vi "CT_SaveMultiWaveformWithNames.vi"(1 "error in (no error)":errorcluster, 2 "delimiter (Tab)":string="\t", 3 "waveforms":waveform(dbl)[][](array[waveform]), 4 "file path (dialog if empty)":path) -> (0 "error out":errorcluster)   [LabVIEW 2009]
panel:
  out "spreadsheet string":string
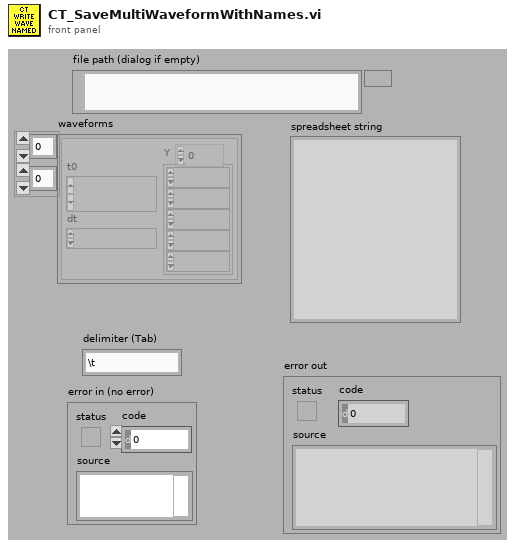
[diagram p1: front panel]
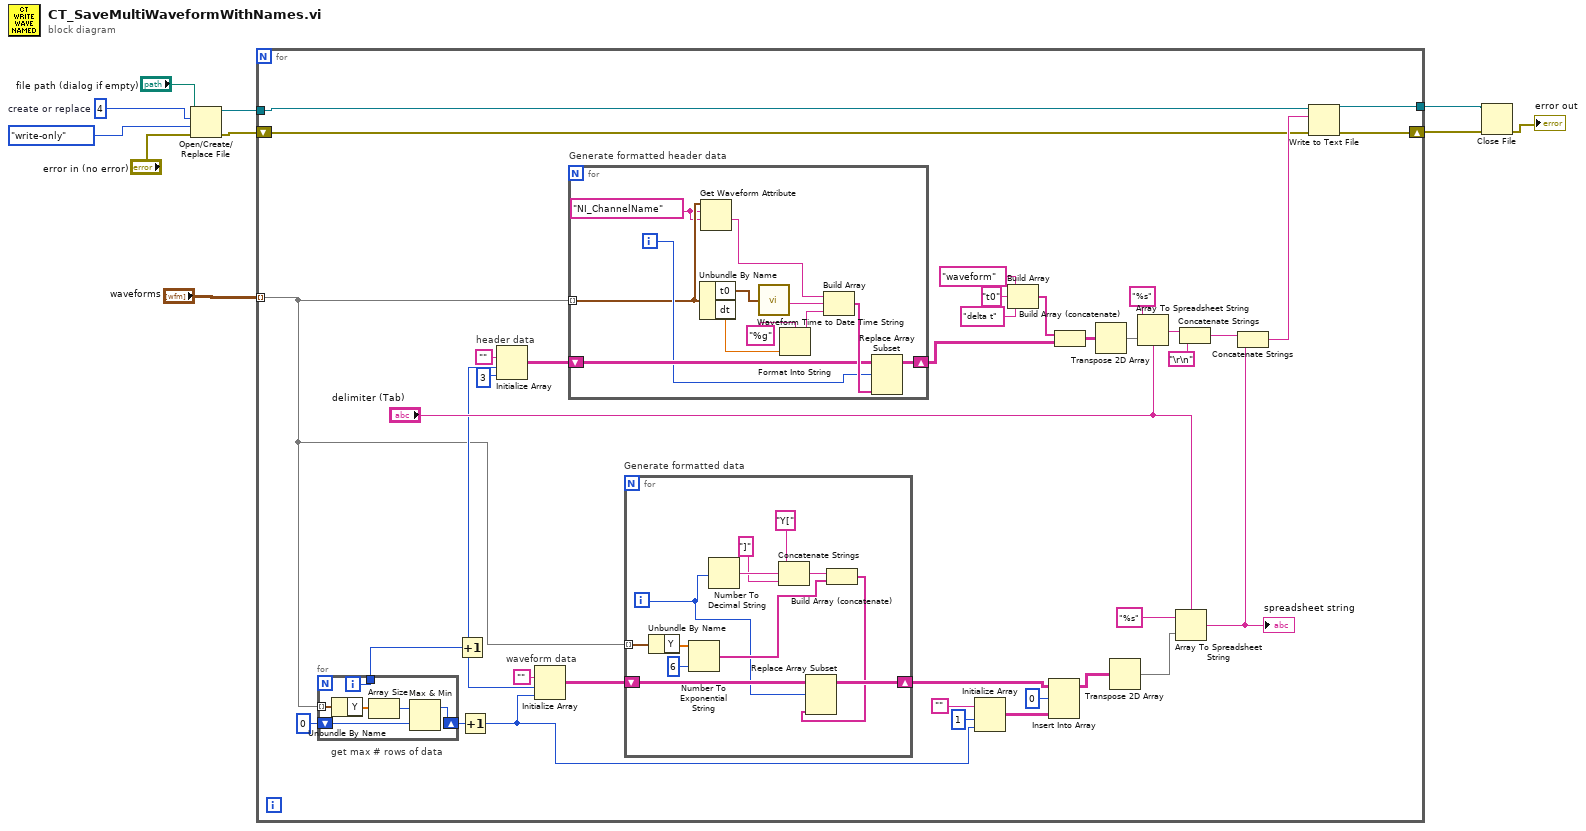
[diagram p0: block diagram]
diagram:
  w5 = i16 4  # create or replace
  n1 = Open/Create/Replace File(file path (use dialog)="file path (dialog if empty)", error in="error in (no error)", operation (0:open)=w5, access (0:read/write)=enum16{"read/write", "read-only", "write-only"}."write-only") -> (refnum out=w3:refnum<file>, error out=w2:errorcluster)  [unwired: 2 in, 1 out]
  n2 = for {
    tunnel: "waveforms" -> [w37] mode=indexing
    tunnel: [w15] -> w9
    tunnel: w3 -> [w12]
    shift-right: [w14] -> w8
    shift-left: w2 -> [w11]
    # "header data"
    # "waveform data"
    # "get max # rows of data"
    n3 = for {
      tunnel: w37 -> [w65] mode=indexing
      shift-right: [w61] -> w41
      shift-left: 0 -> [w62]
      tunnel: [w60] -> w39
      i -> [w60]
      n4 = Unbundle By Name(w65) -> ("Y"=w64:dbl[])
      n5 = Array Size(array=w64) -> (size(s)=w63:i32)
      n6 = Max & Min(x=w63, y=w62) -> (max(x,y)=w61:i32)  [unwired: 1 out]
    }
    n7 = Increment(x=w39) -> (x+1=w38:i32)
    n8 = Increment(x=w41) -> (x+1=w21:i32)
    n9 = Initialize Array("", w38, 3 ("dimension size")) -> (w23:string[][])
    n10 = Initialize Array("", w38, w21) -> (w40:string[][])
    n11 = for "Generate formatted header data" {
      tunnel: w37 -> [w50] mode=indexing
      shift-right: [w52] -> w28
      shift-left: w23 -> [w53]
      i -> [w51]
      w49 = "NI_ChannelName" ("name")
      n12 = Unbundle By Name(w50) -> ("t0"=w55:timestamp, "dt"=w57:dbl)
      n13 = Get Waveform Attribute(5:w49, 6:w49, 7:w50) -> (1:w48:string)  [unwired: 1 in, 3 out]
      n14 = call <vilib>:"Waveform Time to Date Time String.vi"("t0"=w55) -> ("String"=w58:string)
      n15 = Format Into String(format string="%g" ("Format String"), w57) -> (resulting string=w59:string)  [unwired: 2 in, 1 out]
      n16 = Build Array(w48, w58, w59) -> (w54:string[])
      n17 = Replace Array Subset(array=w53, new element=w54, index (row)=w51) -> (w52:string[][])  [unwired: 1 in]
    }
    n18 = for "Generate formatted data" {
      tunnel: w37 -> [w75] mode=indexing
      shift-right: [w73] -> w18
      shift-left: w40 -> [w74]
      i -> [w66]
      n19 = Unbundle By Name(w75) -> ("Y"=w77:dbl[])
      n20 = Number To Exponential String(number=w77, precision (6)=i16 6) -> (E-format string=w72:string[])  [unwired: 2 in]
      n21 = Number To Decimal String(number=w66) -> (decimal integer string=w70:string)  [unwired: 1 in]
      n22 = Concatenate Strings("Y[", w70, "]") -> (w67:string)
      n23 = Build Array (concatenate)(w67, w72) -> (w71:string[])
      n24 = Replace Array Subset(array=w74, new element=w71, index (row)=w66) -> (w73:string[][])  [unwired: 1 in]
    }
    n25 = Initialize Array("", 1 ("dimension size"), w21) -> (w19:string[][])
    n26 = Build Array("waveform", "t0", "delta t") -> (w29:string[])
    n27 = Insert Into Array(array=w18, index (row)=0, new element=w19) -> (w17:string[][])  [unwired: 1 in]
    n28 = Build Array (concatenate)(w29, w28) -> (w26:string[][])
    n29 = Transpose 2D Array(2D array=w26) -> (transposed array=w27:string[][])
    n30 = Transpose 2D Array(2D array=w17) -> (transposed array=w36:string[][])
    n31 = Array To Spreadsheet String(delimiter (Tab)="delimiter (Tab)", array=w27, 3:"%s" ("format string")) -> (spreadsheet string=w31:string)
    n32 = Array To Spreadsheet String(delimiter (Tab)="delimiter (Tab)", array=w36, 3:"%s" ("format (%.3f)")) -> (spreadsheet string=w45:string)
    "spreadsheet string" <- w45
    n33 = Concatenate Strings(w31, "\r\n") -> (w44:string)
    n34 = Concatenate Strings(w44, w45) -> (w13:string)
    n35 = Write to Text File(file (use dialog)=w12, text=w13, error in=w11) -> (refnum out=w15:refnum<file>, error out=w14:errorcluster)  [unwired: 1 in, 1 out]
  }
  n36 = Close File(refnum=w9, error in=w8) -> (error out=→"error out":errorcluster)  [unwired: 1 out]
